vi "Servo Controlled by Accelerometer Example 3.vi"(8 "error in":errorcluster) -> (0 "Error Out":errorcluster)   [LabVIEW 2014]
uses:
  LabVIEW-Universal-Transcriptor-ServoLibrary/ServoDatatype.lvclass
  <vilib>/LabVIEW Universal Transcriptor/LabVIEW to Arduino Transcriptor/Transcriptors/System API/Serial println string.vi
  LabVIEW-Universal-Transcriptor-MPU6050-Library/Arduino MPU6050.lvlib
  <vilib>/LabVIEW Universal Transcriptor/LabVIEW for Arduino Math Library/Arduino Math.lvlib
panel:
  # "Rotates servo motor based on Z-axis acceleration from MPU6050."
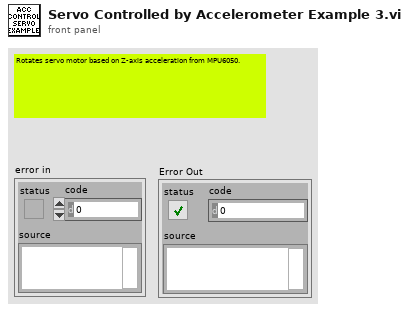
[diagram p1: front panel]
types:
  T1 = enum16{"MPU6050_RANGE_2G", "MPU6050_RANGE_4G", "MPU6050_RANGE_8G", "MPU6050_RANGE_16G"}
  T2 = enum16{"MPU6050_SCALE_250DPS", "MPU6050_SCALE_500DPS", "MPU6050_SCALE_1000DPS", "MPU6050_SCALE_2000DPS"}
  T3 = typedef "Arduino MPU6050.lvlib/Vector.ctl" = cluster{"XAxis":sgl, "YAxis":sgl, "ZAxis":sgl}
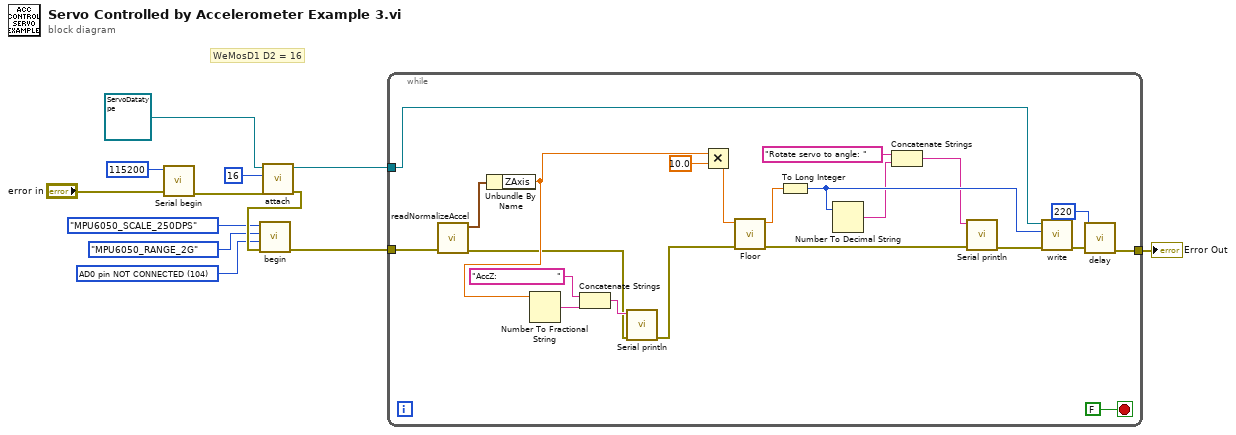
[diagram p0: block diagram]
diagram:
  w4 = u16 104 items=["AD0 pin NOT CONNECTED"=104, "AD0 connect to Vcc"=105] ("address")
  # "WeMosD1 D2 = 16"
  n1 = call <vilib>:"Serial begin.vi"("Error In"="error in", "speed (Bd)"=115200) -> ("Error Out"=w8:errorcluster)  [unwired: 9 in]
  n2 = call-dynamic "attach.vi"("error in (no error)"=w8, "pin number"=16, "Servo in"=refnum<class "ServoDatatype.lvclass"> refnum) -> ("error out"=w10:errorcluster, "Servo out"=w2:refnum<class "ServoDatatype.lvclass">)  [unwired: 6 in, 1 out]
  n3 = call <vilib>:"begin.vi"("Error In"=w10, "address"=w4, "range"=T1."MPU6050_RANGE_2G", "scale"=T2."MPU6050_SCALE_250DPS") -> ("Error Out"=w3:errorcluster)  [unwired: 7 in]
  n4 = while {
    tunnel: w3 -> [w34]
    tunnel: w2 -> [w28]
    tunnel: [w21] -> w1
    stop <- FALSE stop-if-true
    n5 = call <vilib>:"readNormalizeAccel.vi"("error in (no error)"=w34) -> ("error out"=w15:errorcluster, "Vector"=w32:T3)  [unwired: 9 in]
    n6 = Unbundle By Name(w32) -> ("ZAxis"=w16:sgl)
    n7 = Number To Fractional String(number=w16) -> (F-format string=w19:string)  [unwired: 3 in]
    n8 = Concatenate Strings("AccZ:                    " ("string"), w19) -> (w17:string)
    n9 = call-poly <vilib>:"Serial println.vi"("Error In"=w15, "string in"=w17) -> ("Error Out"=w14:errorcluster)  [unwired: 9 in]
    n10 = Multiply(x=w16, y=sgl 10.0) -> (x*y=w31:sgl)
    n11 = call <vilib>:"Floor.vi"("Error In"=w14, "x"=w31) -> ("Error Out"=w30:errorcluster, "floor(x)"=w27:sgl)  [unwired: 8 in]
    n12 = To Long Integer(number=w27) -> (32bit integer=w26:i32)
    n13 = Number To Decimal String(number=w26) -> (decimal integer string=w25:string)  [unwired: 1 in]
    n14 = Concatenate Strings("Rotate servo to angle: " ("string"), w25) -> (w24:string)
    n15 = call-poly <vilib>:"Serial println.vi"("Error In"=w30, "string in"=w24) -> ("Error Out"=w29:errorcluster)  [unwired: 9 in]
    n16 = call-dynamic "write.vi"("error in (no error)"=w29, "value"=w26, "ServoDatatype in"=w28) -> ("error out"=w22:errorcluster)  [unwired: 7 in, 1 out]
    n17 = call <vilib>:"delay.vi"("Error In"=w22, "time (ms)"=220) -> ("Error Out"=w21:errorcluster)  [unwired: 9 in]
  }
  "Error Out" <- w1
